vi "Write Device Information to XML.vi"(8 "error in (no error)":errorcluster, 10 "Device Information":T1[](array[typedef]), 11 "XML Handler in":refnum<class "XML Handler.lvclass">) -> (0 "error out":errorcluster, 3 "XML Handler out":refnum<class "XML Handler.lvclass">)   [LabVIEW 2020, in "XML Handler.lvclass"]
doc: "Writes the device information to the XML file"
uses:
  XML Handler.lvclass
  Devices/Controls/Device Information Cluster.ctl
  Devices/Controls/Register to Write.ctl
  XML Handler.lvclass/XML Handler.ctl
  <vilib>/xml/Close Reference(Node).vi
  <resource>/objmgr/DOMUserDefRef.rc
  <vilib>/xml/NI_XML.lvlib
  Devices/PIC-device/PIC-Device.lvclass
  Devices/Device.lvclass
panel:
  out "Node Value":string
  out "Node Type":i32(ring)=1 items=["Element_Node"=1, "Attribute_Node"=2, "Text_Node"=3, "CDATASection_Node"=4, "EntityReference_Node"=5, "Entity_Node"=6, "ProcessingInstruction_Node"=7, "Comment_Node"=8, "Document_Node"=9, "DocumentType_Node"=10, "DocumentFragment_Node"=11, "Notation_Node"=12]
  out "Node":refnum<k20>
  out "Node Name 2":string
  out "Node Name":string
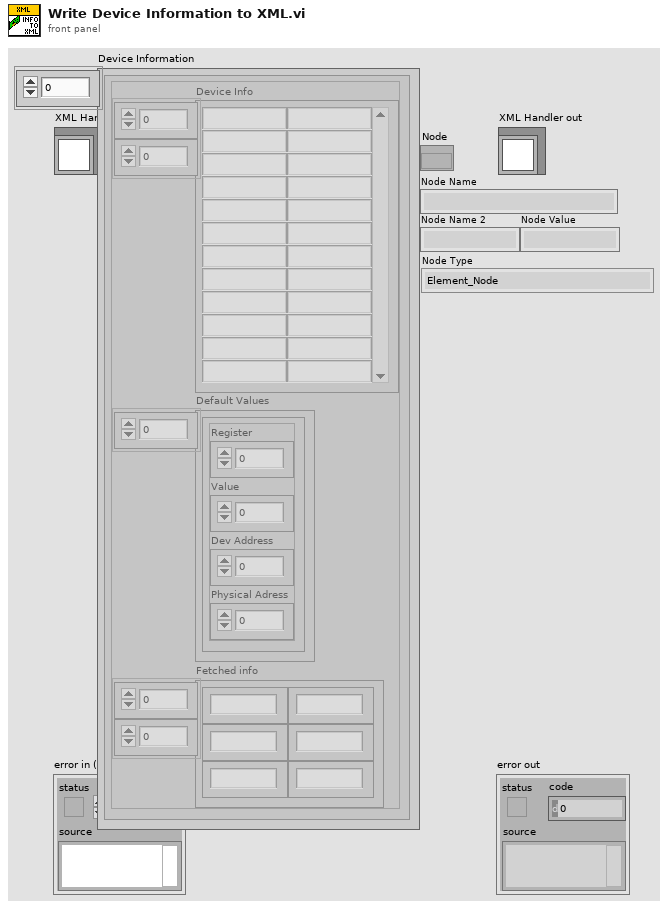
[diagram p1: front panel]
types:
  T1 = typedef "Device.lvclass/Device Information Cluster.ctl" = cluster{"Device Info":string[][], "Default Values":T2[], "Fetched info":string[][]}
  T2 = typedef "PIC-Device.lvclass/Register to Write.ctl" = cluster{"Register":u32, "Value":u32, "Dev Address":u32, "Physical Adress":u32}
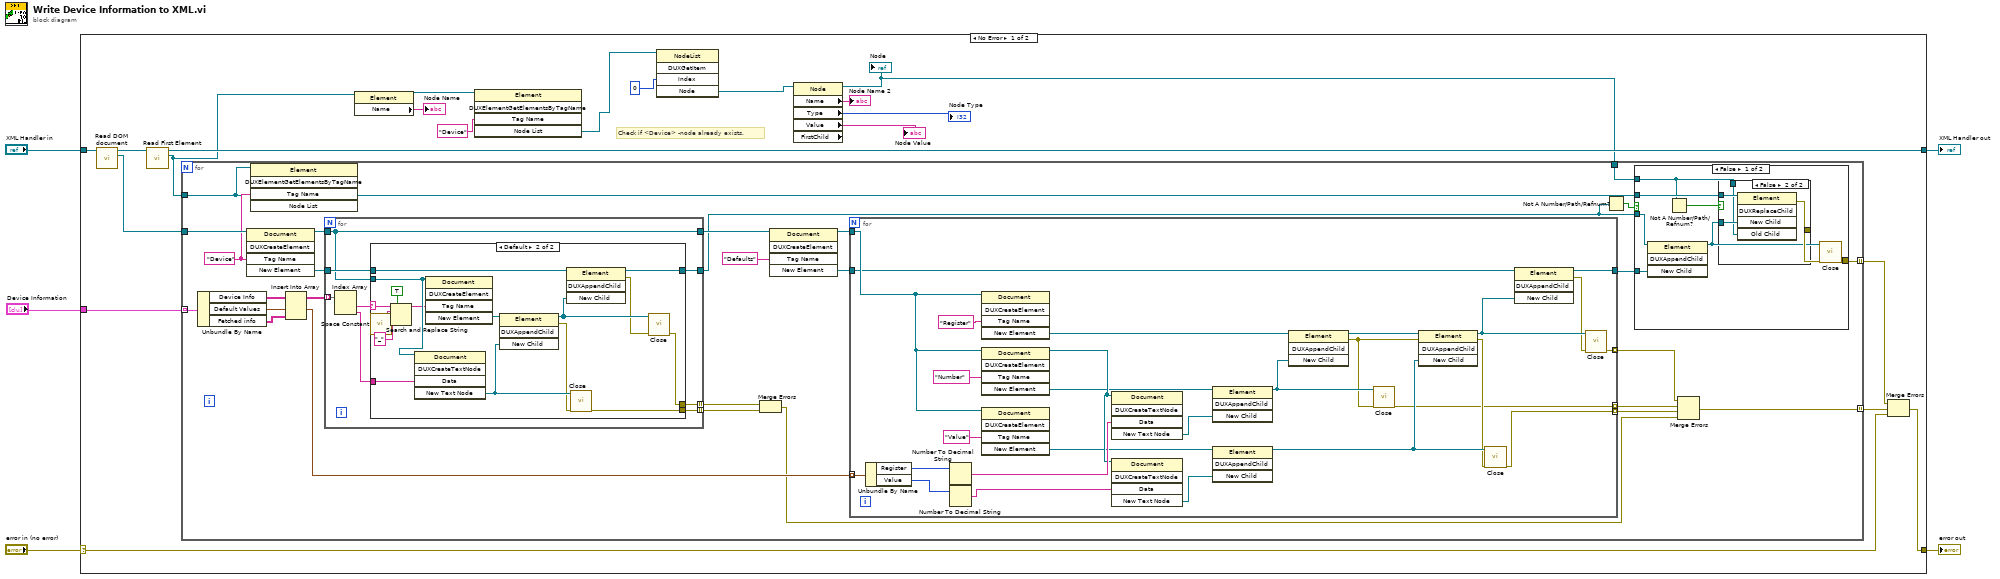
[diagram p0: block diagram]
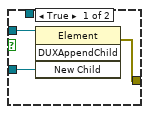
[diagram p2: hidden frame]
diagram:
  n1 = case shown="No Error" "error in (no error)" {
    selector: "error in (no error)" -> [w19 w120]
    tunnel: [w18 w120] -> w4
    tunnel: [w23 w119] -> w2
    tunnel: "XML Handler in" -> [w24 w119]
    tunnel: "Device Information" -> [w22 _]
    frame No Error {
      # "Check if <Device> -node already exists."
      n2 = call "Read DOM document.vi"("XML Handler in"=w24) -> ("DOM document"=w17:refnum<k20>, "XML Handler out"=w25:refnum<class "XML Handler.lvclass">)  [unwired: 9 in]
      n3 = call "Read First Element.vi"("XML Handler in"=w25) -> ("First Element"=w15:refnum<k20>, "XML Handler out"=w23:refnum<class "XML Handler.lvclass">)  [unwired: 9 in]
      n4 = property class="Element"(reference=w15) -> (reference out=w14:refnum<k20>, "Name"=→"Node Name":string)  [unwired: 1 in, 1 out]
      n5 = invoke class="Element" method="DUXElementGetElementsByTagName"(reference=w14, "Tag Name"="Device") -> ("Node List"=w12:refnum<k20>)  [unwired: 3 in, 4 out]
      n6 = invoke class="NodeList" method="DUXGetItem"(reference=w12, "Index"=0) -> ("Node"=w11:refnum<k20>)  [unwired: 3 in, 4 out]
      n7 = property class="Node" props=["Name", "Type", "Value", "FirstChild"](reference=w11) -> (reference out=w6:refnum<k20>, "Name"=→"Node Name 2":string, "Type"=→"Node Type":i32, "Value"=→"Node Value":string)  [unwired: 1 in, 2 out]
      "Node" <- w6
      n8 = for {
        tunnel: w22 -> [w51] mode=indexing
        tunnel: w17 -> [w32]
        tunnel: w15 -> [w29]
        tunnel: [w37] -> w21 mode=indexing
        tunnel: [w36] -> w20 mode=indexing
        tunnel: w6 -> [w26]
        w31 = "Device" ("Tag Name")
        n9 = Unbundle By Name(w51) -> ("Device Info"=w35:string[][], "Default Values"=w46:T2[], "Fetched info"=w33:string[][])
        n10 = invoke class="Document" method="DUXCreateElement"(reference=w32, "Tag Name"=w31) -> (reference out=w50:refnum<k20>, "New Element"=w30:refnum<k20>)  [unwired: 3 in, 3 out]
        n11 = invoke class="Element" method="DUXElementGetElementsByTagName"(reference=w29, "Tag Name"=w31) -> ()  [unwired: 3 in, 5 out]
        n12 = Insert Into Array(array=w35, new element=w33) -> (w34:string[][])  [unwired: 2 in]
        n13 = for {
          tunnel: w50 -> [w99]
          tunnel: w30 -> [w101]
          tunnel: [w100] -> w28
          tunnel: [w99] -> w49
          tunnel: w34 -> [w98] mode=indexing
          tunnel: [w96] -> w43 mode=indexing
          tunnel: [w95] -> w42 mode=indexing
          n14 = Index Array(array=w98) -> (element #1=w94:string, element #2=w97:string)  [unwired: 2 in]
          n15 = case shown="Default" w94 {
            selector: w94 -> [_ w103]
            tunnel: w101 -> [w102 w118]
            tunnel: [w102 w112] -> w100
            tunnel: w99 -> [_ w111]
            tunnel: w97 -> [_ w110]
            tunnel: [_ w105] -> w96
            tunnel: [_ w104] -> w95
            frame "" {
            }
            frame Default {
              n16 = call <vilib>:"Space Constant.vi"() -> ("String"=w109:string)
              n17 = Search and Replace String(replace all?=TRUE ("replace all? (F)"), input string=w103, search string=w109, replace string="_") -> (result string=w106:string)  [unwired: 4 in, 3 out]
              n18 = invoke class="Document" method="DUXCreateTextNode"(reference=w111, "Data"=w110) -> ("New Text Node"=w116:refnum<k20>)  [unwired: 3 in, 4 out]
              n19 = invoke class="Document" method="DUXCreateElement"(reference=w111, "Tag Name"=w106) -> ("New Element"=w117:refnum<k20>)  [unwired: 3 in, 4 out]
              n20 = invoke class="Element" method="DUXAppendChild"(reference=w117, "New Child"=w116) -> (reference out=w114:refnum<k20>, error out=w115:errorcluster)  [unwired: 2 in, 2 out]
              n21 = invoke class="Element" method="DUXAppendChild"(reference=w118, "New Child"=w114) -> (reference out=w112:refnum<k20>, error out=w113:errorcluster)  [unwired: 2 in, 2 out]
              n22 = call-poly <vilib>:"Close.vi"("error in (no error)"=w115, "node"=w116) -> ("error out"=w104:errorcluster)  [unwired: 7 in]
              n23 = call-poly <vilib>:"Close.vi"("error in (no error)"=w113, "node"=w114) -> ("error out"=w105:errorcluster)  [unwired: 7 in]
            }
          }
        }
        n24 = Merge Errors(w43, w42) -> (w41:errorcluster)
        n25 = invoke class="Document" method="DUXCreateElement"(reference=w49, "Tag Name"="Defaults") -> (reference out=w47:refnum<k20>, "New Element"=w45:refnum<k20>)  [unwired: 3 in, 3 out]
        n26 = for {
          tunnel: w47 -> [w90]
          tunnel: w46 -> [w93] mode=indexing
          tunnel: w45 -> [w74]
          tunnel: [w71] -> w44
          tunnel: [w70] -> w40 mode=indexing
          tunnel: [w68] -> w39 mode=indexing
          tunnel: [w67] -> w38 mode=indexing
          n27 = Unbundle By Name(w93) -> ("Register"=w88:u32, "Value"=w85:u32)
          n28 = Number To Decimal String(number=w88) -> (decimal integer string=w87:string)  [unwired: 1 in]
          n29 = Number To Decimal String(number=w85) -> (decimal integer string=w84:string)  [unwired: 1 in]
          n30 = invoke class="Document" method="DUXCreateElement"(reference=w90, "Tag Name"="Register") -> ("New Element"=w83:refnum<k20>)  [unwired: 3 in, 4 out]
          n31 = invoke class="Document" method="DUXCreateElement"(reference=w90, "Tag Name"="Number") -> (reference out=w86:refnum<k20>, "New Element"=w82:refnum<k20>)  [unwired: 3 in, 3 out]
          n32 = invoke class="Document" method="DUXCreateElement"(reference=w90, "Tag Name"="Value") -> ("New Element"=w80:refnum<k20>)  [unwired: 3 in, 4 out]
          n33 = invoke class="Document" method="DUXCreateTextNode"(reference=w86, "Data"=w87) -> ("New Text Node"=w81:refnum<k20>)  [unwired: 3 in, 4 out]
          n34 = invoke class="Document" method="DUXCreateTextNode"(reference=w86, "Data"=w84) -> ("New Text Node"=w79:refnum<k20>)  [unwired: 3 in, 4 out]
          n35 = invoke class="Element" method="DUXAppendChild"(reference=w82, "New Child"=w81) -> (reference out=w78:refnum<k20>)  [unwired: 2 in, 3 out]
          n36 = invoke class="Element" method="DUXAppendChild"(reference=w80, "New Child"=w79) -> (reference out=w76:refnum<k20>)  [unwired: 2 in, 3 out]
          n37 = invoke class="Element" method="DUXAppendChild"(reference=w83, "New Child"=w78) -> (reference out=w77:refnum<k20>, error out=w69:errorcluster)  [unwired: 2 in, 2 out]
          n38 = call-poly <vilib>:"Close.vi"("error in (no error)"=w69, "node"=w78) -> ("error out"=w68:errorcluster)  [unwired: 7 in]
          n39 = invoke class="Element" method="DUXAppendChild"(reference=w77, error in=w69, "New Child"=w76) -> (reference out=w73:refnum<k20>, error out=w75:errorcluster)  [unwired: 1 in, 2 out]
          n40 = call-poly <vilib>:"Close.vi"("error in (no error)"=w75, "node"=w76) -> ("error out"=w70:errorcluster)  [unwired: 7 in]
          n41 = invoke class="Element" method="DUXAppendChild"(reference=w74, "New Child"=w73) -> (reference out=w71:refnum<k20>, error out=w72:errorcluster)  [unwired: 2 in, 2 out]
          n42 = call-poly <vilib>:"Close.vi"("error in (no error)"=w72, "node"=w73) -> ("error out"=w67:errorcluster)  [unwired: 7 in]
        }
        n43 = Not A Number/Path/Refnum?(number/path/refnum=w28) -> (NaN/Path/Refnum?=w27:bool)
        n44 = case shown="False" w27 {
          tunnel: w44 -> [w59 _]
          tunnel: [w57 _] -> w36
          tunnel: w29 -> [w56 _]
          tunnel: w28 -> [w55 _]
          tunnel: w26 -> [w53 _]
          frame False {
            n45 = invoke class="Element" method="DUXAppendChild"(reference=w55, "New Child"=w59) -> (reference out=w54:refnum<k20>)  [unwired: 2 in, 3 out]
            n46 = Not A Number/Path/Refnum?(number/path/refnum=w53) -> (NaN/Path/Refnum?=w52:bool)
            n47 = case shown="False" w52 {
              tunnel: w54 -> [w62 w66]
              tunnel: [w61 w65] -> w58
              tunnel: w56 -> [w60 w64]
              tunnel: w53 -> [_ w63]
              frame True {
                n48 = invoke class="Element" method="DUXAppendChild"(reference=w60, "New Child"=w62) -> (error out=w61:errorcluster)  [unwired: 2 in, 3 out]
              }
              frame False {
                n49 = invoke class="Element" method="DUXReplaceChild"(reference=w64, "New Child"=w66, "Old Child"=w63) -> (error out=w65:errorcluster)  [unwired: 2 in, 4 out]
              }
            }
            n50 = call-poly <vilib>:"Close.vi"("error in (no error)"=w58, "node"=w54) -> ("error out"=w57:errorcluster)  [unwired: 7 in]
          }
          frame True {
          }
        }
        n51 = Merge Errors(w38, w39, w40, w41) -> (w37:errorcluster)
      }
      n52 = Merge Errors(w20, w21, w19) -> (w18:errorcluster)
    }
    frame Error {
    }
  }
  "error out" <- w4
  "XML Handler out" <- w2
